vi "Change_trigger_state.vi"(8 "error in (no error)":errorcluster, 10 "Enable Trigger?":bool, 11 "Control_card in":refnum<class "Control_card.lvclass">) -> (0 "error out":errorcluster, 3 "Control_card out":refnum<class "Control_card.lvclass">)   [LabVIEW 2015, in "Control_card.lvclass"]
uses:
  Control_card.lvclass
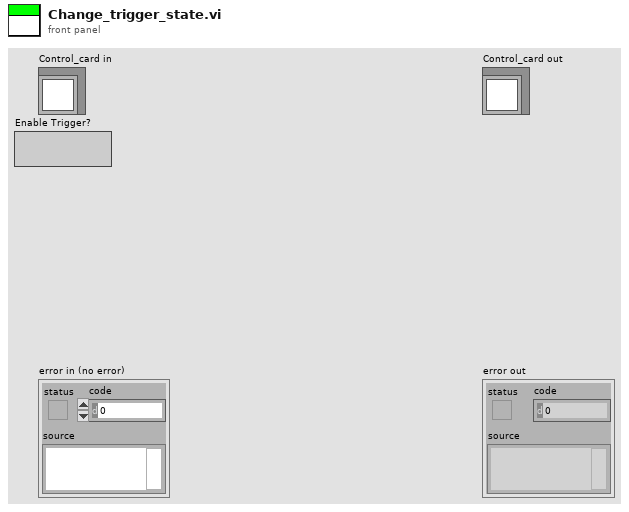
[diagram p1: front panel]
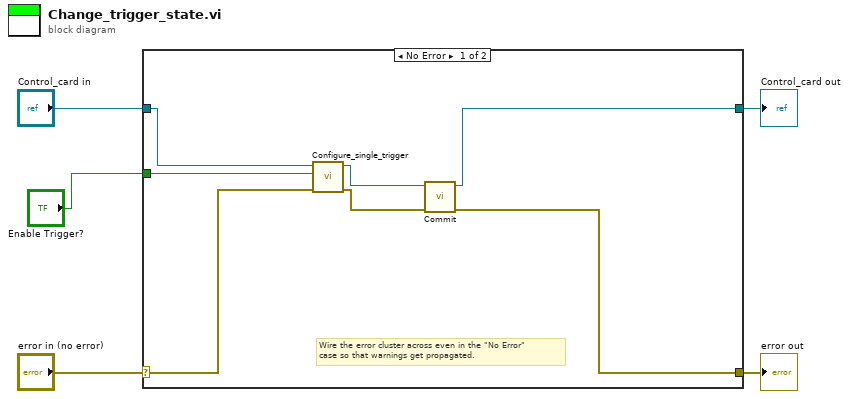
[diagram p0: block diagram]
diagram:
  n1 = case shown="No Error" "error in (no error)" {
    selector: "error in (no error)" -> [w9 w14]
    tunnel: [w7 w14] -> w4
    tunnel: [w6 w13] -> w2
    tunnel: "Control_card in" -> [w12 w13]
    tunnel: "Enable Trigger?" -> [w10 _]
    frame No Error {
      # "Wire the error cluster across even in the \"No Error\"\ncase so that warnings get propagated."
      n2 = call-dynamic "Configure_single_trigger.vi"("error in (no error)"=w9, "Enable Trigger?"=w10, "Initialize_card in"=w12) -> ("error out"=w8:errorcluster, "Initialize_card out"=w11:refnum<class "Control_card.lvclass">)  [unwired: 7 in]
      n3 = call-dynamic "Commit.vi"("error in (no error)"=w8, "Initialize_card in"=w11) -> ("error out"=w7:errorcluster, "Initialize_card out"=w6:refnum<class "Control_card.lvclass">)  [unwired: 8 in]
    }
    frame Error {
    }
  }
  "error out" <- w4
  "Control_card out" <- w2
